vi "良率提醒告知.vi"(0 "Set Count":i32[](array[numeric]), 5 "Use Count":i32[](array[numeric])) -> (3 "String":string, 4 "OverPercentage80":bool=TRUE, 6 "Percentage 80":bool[](array[boolean]), 8 "Percentage100":bool=TRUE, 10 "ArrivePercentage100":bool[](array[boolean]))   [LabVIEW 2019]
uses:
  LLB/Commonly VI/Main Glb.vi
  LLB/Commonly VI.lvlib
panel:
  in  "Blank Button":bool
  out "Array 3":T1[](array[typedef]) items=["0_S1檢平確認氣缸_0", "1_S1檢平確認氣缸_1", "2_S1電路板檢平On次數_0", "3_S1電路板檢平On次數_1", "4_S1 電池檢平On次數_0", "5_S1 電池檢平On次數_1", "6_S1 盒蓋檢平On次數_0", "7_S1 盒蓋檢平On次數_1", "8_S2電流量測探針使用次數_0", "9_S2電流量測探針使用次數_1", "10_S2-電流量測氣缸_0", "11_S2-電流量測氣缸_1", "12_S3程式燒入 探針使用次數_0", "13_S3程式燒入 探針使用次數_1", "14_S3-程式燒入氣缸_0", "15_S3-程式燒入氣缸_1", "16_S4電壓量測探針使用次數_0", "17_S4電壓量測探針使用次數_1", "18_S4電源3V探針使用次數_0", "19_S4電源3V探針使用次數_1", "20_S4-隔離箱上蓋氣缸_0", "21_S4-隔離箱上蓋氣缸_1", "22_S4-隔離箱下蓋氣缸_0", "23_S4-隔離箱下蓋氣缸_1", "24_S4-電池電壓量測固定氣缸_0", "25_S4-電池電壓量測固定氣缸_1", "26_S4-電池電壓量測氣缸_0", "27_S4-電池電壓量測氣缸_1", "28_S4-電路板檢測氣缸_0", "29_S4-電路板檢測氣缸_1", "30_S5-電路板取料升降氣缸_0", "31_S5-電路板取料升降氣缸_1", "32_S5-電路板取料橫移氣缸_0", "33_S5-電路板取料橫移氣缸_1", "34_S5-吸真空_0", "35_S5-吸真空_1", "36_S5-破真空_0", "37_S5-破真空_1", "38_S7-焊接料件固定氣缸_0", "39_S7-焊接料件固定氣缸_1", "40_S7-焊接機清錫馬達_0", "41_S7-焊接機清錫馬達_1", "42_S10-料件翻轉區升降氣缸_0", "43_S10-料件翻轉區升降氣缸_1", "44_S10-料件翻轉區伸出氣缸_0", "45_S10-料件翻轉區伸出氣缸_1", "46_S10-料件翻轉區旋轉氣缸_0", "47_S10-料件翻轉區旋轉氣缸_1", "48_S10-料件翻轉區夾取氣缸_0", "49_S10-料件翻轉區夾取氣缸_1", "50_S10-料件橫移氣缸_0", "51_S10-料件橫移氣缸_1", "52_S10-料件吸取升降氣缸_0", "53_S10-料件吸取升降氣缸_1", "54_S10-料件放料升降氣缸_0", "55_S10-料件放料升降氣缸_1", "56_S10-吸真空_0", "57_S10-吸真空_1", "58_S10-破真空_0", "59_S10-破真空_1", "60_S11-雷射測高檢知氣缸_0", "61_S11-雷射測高檢知氣缸_1", "62_S12-熱熔升降氣缸_0", "63_S12-熱熔升降氣缸_1", "64_S12-預熱升降氣缸_0", "65_S12-預熱升降氣缸_1", "66_S12-離子槍風速調控_0", "67_S12-離子槍風速調控_1", "68_S13-吸真空_0", "69_S13-吸真空_1", "70_S13-破真空_0", "71_S13-破真空_1", "72_S13-NG蓋取料夾爪_0", "73_S13-NG蓋取料夾爪_1", "74_S13-NG蓋取料升降_0", "75_S13-NG蓋取料升降_1", "76_S13-NG電池取料升降_0", "77_S13-NG電池取料升降_1", "78_S13-NG電路板取料升降_0", "79_S13-NG電路板取料升降_1", "80_S13-NG橫移氣缸_0", "81_S13-NG橫移氣缸_1", "82_S13-NG橫移氣缸_0", "83_S13-NG橫移氣缸_1", "84_S7-焊接啟動次數_0", "85_S7-焊接啟動次數_1", "86_S12-熱熔次數_0", "87_S12-熱熔次數_1", "88_S11-雷射檢測次數_0", "89_S11-雷射檢測次數_1"]
  in  "Array 2":enum16{""}[](array[ring])
  out "cluster":T2 {"Array 4[0]" items=["0_S1檢平確認氣缸_0", "1_S1檢平確認氣缸_1", "2_S1電路板檢平On次數_0", "3_S1電路板檢平On次數_1", "4_S1 電池檢平On次數_0", "5_S1 電池檢平On次數_1", "6_S1 盒蓋檢平On次數_0", "7_S1 盒蓋檢平On次數_1", "8_S2電流量測探針使用次數_0", "9_S2電流量測探針使用次數_1", "10_S2-電流量測氣缸_0", "11_S2-電流量測氣缸_1", "12_S3程式燒入 探針使用次數_0", "13_S3程式燒入 探針使用次數_1", "14_S3-程式燒入氣缸_0", "15_S3-程式燒入氣缸_1", "16_S4電壓量測探針使用次數_0", "17_S4電壓量測探針使用次數_1", "18_S4電源3V探針使用次數_0", "19_S4電源3V探針使用次數_1", "20_S4-隔離箱上蓋氣缸_0", "21_S4-隔離箱上蓋氣缸_1", "22_S4-隔離箱下蓋氣缸_0", "23_S4-隔離箱下蓋氣缸_1", "24_S4-電池電壓量測固定氣缸_0", "25_S4-電池電壓量測固定氣缸_1", "26_S4-電池電壓量測氣缸_0", "27_S4-電池電壓量測氣缸_1", "28_S4-電路板檢測氣缸_0", "29_S4-電路板檢測氣缸_1", "30_S5-電路板取料升降氣缸_0", "31_S5-電路板取料升降氣缸_1", "32_S5-電路板取料橫移氣缸_0", "33_S5-電路板取料橫移氣缸_1", "34_S5-吸真空_0", "35_S5-吸真空_1", "36_S5-破真空_0", "37_S5-破真空_1", "38_S7-焊接料件固定氣缸_0", "39_S7-焊接料件固定氣缸_1", "40_S7-焊接機清錫馬達_0", "41_S7-焊接機清錫馬達_1", "42_S10-料件翻轉區升降氣缸_0", "43_S10-料件翻轉區升降氣缸_1", "44_S10-料件翻轉區伸出氣缸_0", "45_S10-料件翻轉區伸出氣缸_1", "46_S10-料件翻轉區旋轉氣缸_0", "47_S10-料件翻轉區旋轉氣缸_1", "48_S10-料件翻轉區夾取氣缸_0", "49_S10-料件翻轉區夾取氣缸_1", "50_S10-料件橫移氣缸_0", "51_S10-料件橫移氣缸_1", "52_S10-料件吸取升降氣缸_0", "53_S10-料件吸取升降氣缸_1", "54_S10-料件放料升降氣缸_0", "55_S10-料件放料升降氣缸_1", "56_S10-吸真空_0", "57_S10-吸真空_1", "58_S10-破真空_0", "59_S10-破真空_1", "60_S11-雷射測高檢知氣缸_0", "61_S11-雷射測高檢知氣缸_1", "62_S12-熱熔升降氣缸_0", "63_S12-熱熔升降氣缸_1", "64_S12-預熱升降氣缸_0", "65_S12-預熱升降氣缸_1", "66_S12-離子槍風速調控_0", "67_S12-離子槍風速調控_1", "68_S13-吸真空_0", "69_S13-吸真空_1", "70_S13-破真空_0", "71_S13-破真空_1", "72_S13-NG蓋取料夾爪_0", "73_S13-NG蓋取料夾爪_1", "74_S13-NG蓋取料升降_0", "75_S13-NG蓋取料升降_1", "76_S13-NG電池取料升降_0", "77_S13-NG電池取料升降_1", "78_S13-NG電路板取料升降_0", "79_S13-NG電路板取料升降_1", "80_S13-NG橫移氣缸_0", "81_S13-NG橫移氣缸_1", "82_S13-NG橫移氣缸_0", "83_S13-NG橫移氣缸_1", "84_S7-焊接啟動次數_0", "85_S7-焊接啟動次數_1", "86_S12-熱熔次數_0", "87_S12-熱熔次數_1", "88_S11-雷射檢測次數_0", "89_S11-雷射檢測次數_1"]; "Array 4[1]" items=["0_S1檢平確認氣缸_0", "1_S1檢平確認氣缸_1", "2_S1電路板檢平On次數_0", "3_S1電路板檢平On次數_1", "4_S1 電池檢平On次數_0", "5_S1 電池檢平On次數_1", "6_S1 盒蓋檢平On次數_0", "7_S1 盒蓋檢平On次數_1", "8_S2電流量測探針使用次數_0", "9_S2電流量測探針使用次數_1", "10_S2-電流量測氣缸_0", "11_S2-電流量測氣缸_1", "12_S3程式燒入 探針使用次數_0", "13_S3程式燒入 探針使用次數_1", "14_S3-程式燒入氣缸_0", "15_S3-程式燒入氣缸_1", "16_S4電壓量測探針使用次數_0", "17_S4電壓量測探針使用次數_1", "18_S4電源3V探針使用次數_0", "19_S4電源3V探針使用次數_1", "20_S4-隔離箱上蓋氣缸_0", "21_S4-隔離箱上蓋氣缸_1", "22_S4-隔離箱下蓋氣缸_0", "23_S4-隔離箱下蓋氣缸_1", "24_S4-電池電壓量測固定氣缸_0", "25_S4-電池電壓量測固定氣缸_1", "26_S4-電池電壓量測氣缸_0", "27_S4-電池電壓量測氣缸_1", "28_S4-電路板檢測氣缸_0", "29_S4-電路板檢測氣缸_1", "30_S5-電路板取料升降氣缸_0", "31_S5-電路板取料升降氣缸_1", "32_S5-電路板取料橫移氣缸_0", "33_S5-電路板取料橫移氣缸_1", "34_S5-吸真空_0", "35_S5-吸真空_1", "36_S5-破真空_0", "37_S5-破真空_1", "38_S7-焊接料件固定氣缸_0", "39_S7-焊接料件固定氣缸_1", "40_S7-焊接機清錫馬達_0", "41_S7-焊接機清錫馬達_1", "42_S10-料件翻轉區升降氣缸_0", "43_S10-料件翻轉區升降氣缸_1", "44_S10-料件翻轉區伸出氣缸_0", "45_S10-料件翻轉區伸出氣缸_1", "46_S10-料件翻轉區旋轉氣缸_0", "47_S10-料件翻轉區旋轉氣缸_1", "48_S10-料件翻轉區夾取氣缸_0", "49_S10-料件翻轉區夾取氣缸_1", "50_S10-料件橫移氣缸_0", "51_S10-料件橫移氣缸_1", "52_S10-料件吸取升降氣缸_0", "53_S10-料件吸取升降氣缸_1", "54_S10-料件放料升降氣缸_0", "55_S10-料件放料升降氣缸_1", "56_S10-吸真空_0", "57_S10-吸真空_1", "58_S10-破真空_0", "59_S10-破真空_1", "60_S11-雷射測高檢知氣缸_0", "61_S11-雷射測高檢知氣缸_1", "62_S12-熱熔升降氣缸_0", "63_S12-熱熔升降氣缸_1", "64_S12-預熱升降氣缸_0", "65_S12-預熱升降氣缸_1", "66_S12-離子槍風速調控_0", "67_S12-離子槍風速調控_1", "68_S13-吸真空_0", "69_S13-吸真空_1", "70_S13-破真空_0", "71_S13-破真空_1", "72_S13-NG蓋取料夾爪_0", "73_S13-NG蓋取料夾爪_1", "74_S13-NG蓋取料升降_0", "75_S13-NG蓋取料升降_1", "76_S13-NG電池取料升降_0", "77_S13-NG電池取料升降_1", "78_S13-NG電路板取料升降_0", "79_S13-NG電路板取料升降_1", "80_S13-NG橫移氣缸_0", "81_S13-NG橫移氣缸_1", "82_S13-NG橫移氣缸_0", "83_S13-NG橫移氣缸_1", "84_S7-焊接啟動次數_0", "85_S7-焊接啟動次數_1", "86_S12-熱熔次數_0", "87_S12-熱熔次數_1", "88_S11-雷射檢測次數_0", "89_S11-雷射檢測次數_1"]; "Array 4[2]" items=["0_S1檢平確認氣缸_0", "1_S1檢平確認氣缸_1", "2_S1電路板檢平On次數_0", "3_S1電路板檢平On次數_1", "4_S1 電池檢平On次數_0", "5_S1 電池檢平On次數_1", "6_S1 盒蓋檢平On次數_0", "7_S1 盒蓋檢平On次數_1", "8_S2電流量測探針使用次數_0", "9_S2電流量測探針使用次數_1", "10_S2-電流量測氣缸_0", "11_S2-電流量測氣缸_1", "12_S3程式燒入 探針使用次數_0", "13_S3程式燒入 探針使用次數_1", "14_S3-程式燒入氣缸_0", "15_S3-程式燒入氣缸_1", "16_S4電壓量測探針使用次數_0", "17_S4電壓量測探針使用次數_1", "18_S4電源3V探針使用次數_0", "19_S4電源3V探針使用次數_1", "20_S4-隔離箱上蓋氣缸_0", "21_S4-隔離箱上蓋氣缸_1", "22_S4-隔離箱下蓋氣缸_0", "23_S4-隔離箱下蓋氣缸_1", "24_S4-電池電壓量測固定氣缸_0", "25_S4-電池電壓量測固定氣缸_1", "26_S4-電池電壓量測氣缸_0", "27_S4-電池電壓量測氣缸_1", "28_S4-電路板檢測氣缸_0", "29_S4-電路板檢測氣缸_1", "30_S5-電路板取料升降氣缸_0", "31_S5-電路板取料升降氣缸_1", "32_S5-電路板取料橫移氣缸_0", "33_S5-電路板取料橫移氣缸_1", "34_S5-吸真空_0", "35_S5-吸真空_1", "36_S5-破真空_0", "37_S5-破真空_1", "38_S7-焊接料件固定氣缸_0", "39_S7-焊接料件固定氣缸_1", "40_S7-焊接機清錫馬達_0", "41_S7-焊接機清錫馬達_1", "42_S10-料件翻轉區升降氣缸_0", "43_S10-料件翻轉區升降氣缸_1", "44_S10-料件翻轉區伸出氣缸_0", "45_S10-料件翻轉區伸出氣缸_1", "46_S10-料件翻轉區旋轉氣缸_0", "47_S10-料件翻轉區旋轉氣缸_1", "48_S10-料件翻轉區夾取氣缸_0", "49_S10-料件翻轉區夾取氣缸_1", "50_S10-料件橫移氣缸_0", "51_S10-料件橫移氣缸_1", "52_S10-料件吸取升降氣缸_0", "53_S10-料件吸取升降氣缸_1", "54_S10-料件放料升降氣缸_0", "55_S10-料件放料升降氣缸_1", "56_S10-吸真空_0", "57_S10-吸真空_1", "58_S10-破真空_0", "59_S10-破真空_1", "60_S11-雷射測高檢知氣缸_0", "61_S11-雷射測高檢知氣缸_1", "62_S12-熱熔升降氣缸_0", "63_S12-熱熔升降氣缸_1", "64_S12-預熱升降氣缸_0", "65_S12-預熱升降氣缸_1", "66_S12-離子槍風速調控_0", "67_S12-離子槍風速調控_1", "68_S13-吸真空_0", "69_S13-吸真空_1", "70_S13-破真空_0", "71_S13-破真空_1", "72_S13-NG蓋取料夾爪_0", "73_S13-NG蓋取料夾爪_1", "74_S13-NG蓋取料升降_0", "75_S13-NG蓋取料升降_1", "76_S13-NG電池取料升降_0", "77_S13-NG電池取料升降_1", "78_S13-NG電路板取料升降_0", "79_S13-NG電路板取料升降_1", "80_S13-NG橫移氣缸_0", "81_S13-NG橫移氣缸_1", "82_S13-NG橫移氣缸_0", "83_S13-NG橫移氣缸_1", "84_S7-焊接啟動次數_0", "85_S7-焊接啟動次數_1", "86_S12-熱熔次數_0", "87_S12-熱熔次數_1", "88_S11-雷射檢測次數_0", "89_S11-雷射檢測次數_1"]; "Array 4[3]" items=["0_S1檢平確認氣缸_0", "1_S1檢平確認氣缸_1", "2_S1電路板檢平On次數_0", "3_S1電路板檢平On次數_1", "4_S1 電池檢平On次數_0", "5_S1 電池檢平On次數_1", "6_S1 盒蓋檢平On次數_0", "7_S1 盒蓋檢平On次數_1", "8_S2電流量測探針使用次數_0", "9_S2電流量測探針使用次數_1", "10_S2-電流量測氣缸_0", "11_S2-電流量測氣缸_1", "12_S3程式燒入 探針使用次數_0", "13_S3程式燒入 探針使用次數_1", "14_S3-程式燒入氣缸_0", "15_S3-程式燒入氣缸_1", "16_S4電壓量測探針使用次數_0", "17_S4電壓量測探針使用次數_1", "18_S4電源3V探針使用次數_0", "19_S4電源3V探針使用次數_1", "20_S4-隔離箱上蓋氣缸_0", "21_S4-隔離箱上蓋氣缸_1", "22_S4-隔離箱下蓋氣缸_0", "23_S4-隔離箱下蓋氣缸_1", "24_S4-電池電壓量測固定氣缸_0", "25_S4-電池電壓量測固定氣缸_1", "26_S4-電池電壓量測氣缸_0", "27_S4-電池電壓量測氣缸_1", "28_S4-電路板檢測氣缸_0", "29_S4-電路板檢測氣缸_1", "30_S5-電路板取料升降氣缸_0", "31_S5-電路板取料升降氣缸_1", "32_S5-電路板取料橫移氣缸_0", "33_S5-電路板取料橫移氣缸_1", "34_S5-吸真空_0", "35_S5-吸真空_1", "36_S5-破真空_0", "37_S5-破真空_1", "38_S7-焊接料件固定氣缸_0", "39_S7-焊接料件固定氣缸_1", "40_S7-焊接機清錫馬達_0", "41_S7-焊接機清錫馬達_1", "42_S10-料件翻轉區升降氣缸_0", "43_S10-料件翻轉區升降氣缸_1", "44_S10-料件翻轉區伸出氣缸_0", "45_S10-料件翻轉區伸出氣缸_1", "46_S10-料件翻轉區旋轉氣缸_0", "47_S10-料件翻轉區旋轉氣缸_1", "48_S10-料件翻轉區夾取氣缸_0", "49_S10-料件翻轉區夾取氣缸_1", "50_S10-料件橫移氣缸_0", "51_S10-料件橫移氣缸_1", "52_S10-料件吸取升降氣缸_0", "53_S10-料件吸取升降氣缸_1", "54_S10-料件放料升降氣缸_0", "55_S10-料件放料升降氣缸_1", "56_S10-吸真空_0", "57_S10-吸真空_1", "58_S10-破真空_0", "59_S10-破真空_1", "60_S11-雷射測高檢知氣缸_0", "61_S11-雷射測高檢知氣缸_1", "62_S12-熱熔升降氣缸_0", "63_S12-熱熔升降氣缸_1", "64_S12-預熱升降氣缸_0", "65_S12-預熱升降氣缸_1", "66_S12-離子槍風速調控_0", "67_S12-離子槍風速調控_1", "68_S13-吸真空_0", "69_S13-吸真空_1", "70_S13-破真空_0", "71_S13-破真空_1", "72_S13-NG蓋取料夾爪_0", "73_S13-NG蓋取料夾爪_1", "74_S13-NG蓋取料升降_0", "75_S13-NG蓋取料升降_1", "76_S13-NG電池取料升降_0", "77_S13-NG電池取料升降_1", "78_S13-NG電路板取料升降_0", "79_S13-NG電路板取料升降_1", "80_S13-NG橫移氣缸_0", "81_S13-NG橫移氣缸_1", "82_S13-NG橫移氣缸_0", "83_S13-NG橫移氣缸_1", "84_S7-焊接啟動次數_0", "85_S7-焊接啟動次數_1", "86_S12-熱熔次數_0", "87_S12-熱熔次數_1", "88_S11-雷射檢測次數_0", "89_S11-雷射檢測次數_1"]; "Array 4[4]" items=["0_S1檢平確認氣缸_0", "1_S1檢平確認氣缸_1", "2_S1電路板檢平On次數_0", "3_S1電路板檢平On次數_1", "4_S1 電池檢平On次數_0", "5_S1 電池檢平On次數_1", "6_S1 盒蓋檢平On次數_0", "7_S1 盒蓋檢平On次數_1", "8_S2電流量測探針使用次數_0", "9_S2電流量測探針使用次數_1", "10_S2-電流量測氣缸_0", "11_S2-電流量測氣缸_1", "12_S3程式燒入 探針使用次數_0", "13_S3程式燒入 探針使用次數_1", "14_S3-程式燒入氣缸_0", "15_S3-程式燒入氣缸_1", "16_S4電壓量測探針使用次數_0", "17_S4電壓量測探針使用次數_1", "18_S4電源3V探針使用次數_0", "19_S4電源3V探針使用次數_1", "20_S4-隔離箱上蓋氣缸_0", "21_S4-隔離箱上蓋氣缸_1", "22_S4-隔離箱下蓋氣缸_0", "23_S4-隔離箱下蓋氣缸_1", "24_S4-電池電壓量測固定氣缸_0", "25_S4-電池電壓量測固定氣缸_1", "26_S4-電池電壓量測氣缸_0", "27_S4-電池電壓量測氣缸_1", "28_S4-電路板檢測氣缸_0", "29_S4-電路板檢測氣缸_1", "30_S5-電路板取料升降氣缸_0", "31_S5-電路板取料升降氣缸_1", "32_S5-電路板取料橫移氣缸_0", "33_S5-電路板取料橫移氣缸_1", "34_S5-吸真空_0", "35_S5-吸真空_1", "36_S5-破真空_0", "37_S5-破真空_1", "38_S7-焊接料件固定氣缸_0", "39_S7-焊接料件固定氣缸_1", "40_S7-焊接機清錫馬達_0", "41_S7-焊接機清錫馬達_1", "42_S10-料件翻轉區升降氣缸_0", "43_S10-料件翻轉區升降氣缸_1", "44_S10-料件翻轉區伸出氣缸_0", "45_S10-料件翻轉區伸出氣缸_1", "46_S10-料件翻轉區旋轉氣缸_0", "47_S10-料件翻轉區旋轉氣缸_1", "48_S10-料件翻轉區夾取氣缸_0", "49_S10-料件翻轉區夾取氣缸_1", "50_S10-料件橫移氣缸_0", "51_S10-料件橫移氣缸_1", "52_S10-料件吸取升降氣缸_0", "53_S10-料件吸取升降氣缸_1", "54_S10-料件放料升降氣缸_0", "55_S10-料件放料升降氣缸_1", "56_S10-吸真空_0", "57_S10-吸真空_1", "58_S10-破真空_0", "59_S10-破真空_1", "60_S11-雷射測高檢知氣缸_0", "61_S11-雷射測高檢知氣缸_1", "62_S12-熱熔升降氣缸_0", "63_S12-熱熔升降氣缸_1", "64_S12-預熱升降氣缸_0", "65_S12-預熱升降氣缸_1", "66_S12-離子槍風速調控_0", "67_S12-離子槍風速調控_1", "68_S13-吸真空_0", "69_S13-吸真空_1", "70_S13-破真空_0", "71_S13-破真空_1", "72_S13-NG蓋取料夾爪_0", "73_S13-NG蓋取料夾爪_1", "74_S13-NG蓋取料升降_0", "75_S13-NG蓋取料升降_1", "76_S13-NG電池取料升降_0", "77_S13-NG電池取料升降_1", "78_S13-NG電路板取料升降_0", "79_S13-NG電路板取料升降_1", "80_S13-NG橫移氣缸_0", "81_S13-NG橫移氣缸_1", "82_S13-NG橫移氣缸_0", "83_S13-NG橫移氣缸_1", "84_S7-焊接啟動次數_0", "85_S7-焊接啟動次數_1", "86_S12-熱熔次數_0", "87_S12-熱熔次數_1", "88_S11-雷射檢測次數_0", "89_S11-雷射檢測次數_1"]; "Array 4[5]" items=["0_S1檢平確認氣缸_0", "1_S1檢平確認氣缸_1", "2_S1電路板檢平On次數_0", "3_S1電路板檢平On次數_1", "4_S1 電池檢平On次數_0", "5_S1 電池檢平On次數_1", "6_S1 盒蓋檢平On次數_0", "7_S1 盒蓋檢平On次數_1", "8_S2電流量測探針使用次數_0", "9_S2電流量測探針使用次數_1", "10_S2-電流量測氣缸_0", "11_S2-電流量測氣缸_1", "12_S3程式燒入 探針使用次數_0", "13_S3程式燒入 探針使用次數_1", "14_S3-程式燒入氣缸_0", "15_S3-程式燒入氣缸_1", "16_S4電壓量測探針使用次數_0", "17_S4電壓量測探針使用次數_1", "18_S4電源3V探針使用次數_0", "19_S4電源3V探針使用次數_1", "20_S4-隔離箱上蓋氣缸_0", "21_S4-隔離箱上蓋氣缸_1", "22_S4-隔離箱下蓋氣缸_0", "23_S4-隔離箱下蓋氣缸_1", "24_S4-電池電壓量測固定氣缸_0", "25_S4-電池電壓量測固定氣缸_1", "26_S4-電池電壓量測氣缸_0", "27_S4-電池電壓量測氣缸_1", "28_S4-電路板檢測氣缸_0", "29_S4-電路板檢測氣缸_1", "30_S5-電路板取料升降氣缸_0", "31_S5-電路板取料升降氣缸_1", "32_S5-電路板取料橫移氣缸_0", "33_S5-電路板取料橫移氣缸_1", "34_S5-吸真空_0", "35_S5-吸真空_1", "36_S5-破真空_0", "37_S5-破真空_1", "38_S7-焊接料件固定氣缸_0", "39_S7-焊接料件固定氣缸_1", "40_S7-焊接機清錫馬達_0", "41_S7-焊接機清錫馬達_1", "42_S10-料件翻轉區升降氣缸_0", "43_S10-料件翻轉區升降氣缸_1", "44_S10-料件翻轉區伸出氣缸_0", "45_S10-料件翻轉區伸出氣缸_1", "46_S10-料件翻轉區旋轉氣缸_0", "47_S10-料件翻轉區旋轉氣缸_1", "48_S10-料件翻轉區夾取氣缸_0", "49_S10-料件翻轉區夾取氣缸_1", "50_S10-料件橫移氣缸_0", "51_S10-料件橫移氣缸_1", "52_S10-料件吸取升降氣缸_0", "53_S10-料件吸取升降氣缸_1", "54_S10-料件放料升降氣缸_0", "55_S10-料件放料升降氣缸_1", "56_S10-吸真空_0", "57_S10-吸真空_1", "58_S10-破真空_0", "59_S10-破真空_1", "60_S11-雷射測高檢知氣缸_0", "61_S11-雷射測高檢知氣缸_1", "62_S12-熱熔升降氣缸_0", "63_S12-熱熔升降氣缸_1", "64_S12-預熱升降氣缸_0", "65_S12-預熱升降氣缸_1", "66_S12-離子槍風速調控_0", "67_S12-離子槍風速調控_1", "68_S13-吸真空_0", "69_S13-吸真空_1", "70_S13-破真空_0", "71_S13-破真空_1", "72_S13-NG蓋取料夾爪_0", "73_S13-NG蓋取料夾爪_1", "74_S13-NG蓋取料升降_0", "75_S13-NG蓋取料升降_1", "76_S13-NG電池取料升降_0", "77_S13-NG電池取料升降_1", "78_S13-NG電路板取料升降_0", "79_S13-NG電路板取料升降_1", "80_S13-NG橫移氣缸_0", "81_S13-NG橫移氣缸_1", "82_S13-NG橫移氣缸_0", "83_S13-NG橫移氣缸_1", "84_S7-焊接啟動次數_0", "85_S7-焊接啟動次數_1", "86_S12-熱熔次數_0", "87_S12-熱熔次數_1", "88_S11-雷射檢測次數_0", "89_S11-雷射檢測次數_1"]; "Array 4[6]" items=["0_S1檢平確認氣缸_0", "1_S1檢平確認氣缸_1", "2_S1電路板檢平On次數_0", "3_S1電路板檢平On次數_1", "4_S1 電池檢平On次數_0", "5_S1 電池檢平On次數_1", "6_S1 盒蓋檢平On次數_0", "7_S1 盒蓋檢平On次數_1", "8_S2電流量測探針使用次數_0", "9_S2電流量測探針使用次數_1", "10_S2-電流量測氣缸_0", "11_S2-電流量測氣缸_1", "12_S3程式燒入 探針使用次數_0", "13_S3程式燒入 探針使用次數_1", "14_S3-程式燒入氣缸_0", "15_S3-程式燒入氣缸_1", "16_S4電壓量測探針使用次數_0", "17_S4電壓量測探針使用次數_1", "18_S4電源3V探針使用次數_0", "19_S4電源3V探針使用次數_1", "20_S4-隔離箱上蓋氣缸_0", "21_S4-隔離箱上蓋氣缸_1", "22_S4-隔離箱下蓋氣缸_0", "23_S4-隔離箱下蓋氣缸_1", "24_S4-電池電壓量測固定氣缸_0", "25_S4-電池電壓量測固定氣缸_1", "26_S4-電池電壓量測氣缸_0", "27_S4-電池電壓量測氣缸_1", "28_S4-電路板檢測氣缸_0", "29_S4-電路板檢測氣缸_1", "30_S5-電路板取料升降氣缸_0", "31_S5-電路板取料升降氣缸_1", "32_S5-電路板取料橫移氣缸_0", "33_S5-電路板取料橫移氣缸_1", "34_S5-吸真空_0", "35_S5-吸真空_1", "36_S5-破真空_0", "37_S5-破真空_1", "38_S7-焊接料件固定氣缸_0", "39_S7-焊接料件固定氣缸_1", "40_S7-焊接機清錫馬達_0", "41_S7-焊接機清錫馬達_1", "42_S10-料件翻轉區升降氣缸_0", "43_S10-料件翻轉區升降氣缸_1", "44_S10-料件翻轉區伸出氣缸_0", "45_S10-料件翻轉區伸出氣缸_1", "46_S10-料件翻轉區旋轉氣缸_0", "47_S10-料件翻轉區旋轉氣缸_1", "48_S10-料件翻轉區夾取氣缸_0", "49_S10-料件翻轉區夾取氣缸_1", "50_S10-料件橫移氣缸_0", "51_S10-料件橫移氣缸_1", "52_S10-料件吸取升降氣缸_0", "53_S10-料件吸取升降氣缸_1", "54_S10-料件放料升降氣缸_0", "55_S10-料件放料升降氣缸_1", "56_S10-吸真空_0", "57_S10-吸真空_1", "58_S10-破真空_0", "59_S10-破真空_1", "60_S11-雷射測高檢知氣缸_0", "61_S11-雷射測高檢知氣缸_1", "62_S12-熱熔升降氣缸_0", "63_S12-熱熔升降氣缸_1", "64_S12-預熱升降氣缸_0", "65_S12-預熱升降氣缸_1", "66_S12-離子槍風速調控_0", "67_S12-離子槍風速調控_1", "68_S13-吸真空_0", "69_S13-吸真空_1", "70_S13-破真空_0", "71_S13-破真空_1", "72_S13-NG蓋取料夾爪_0", "73_S13-NG蓋取料夾爪_1", "74_S13-NG蓋取料升降_0", "75_S13-NG蓋取料升降_1", "76_S13-NG電池取料升降_0", "77_S13-NG電池取料升降_1", "78_S13-NG電路板取料升降_0", "79_S13-NG電路板取料升降_1", "80_S13-NG橫移氣缸_0", "81_S13-NG橫移氣缸_1", "82_S13-NG橫移氣缸_0", "83_S13-NG橫移氣缸_1", "84_S7-焊接啟動次數_0", "85_S7-焊接啟動次數_1", "86_S12-熱熔次數_0", "87_S12-熱熔次數_1", "88_S11-雷射檢測次數_0", "89_S11-雷射檢測次數_1"]; "Array 4[7]" items=["0_S1檢平確認氣缸_0", "1_S1檢平確認氣缸_1", "2_S1電路板檢平On次數_0", "3_S1電路板檢平On次數_1", "4_S1 電池檢平On次數_0", "5_S1 電池檢平On次數_1", "6_S1 盒蓋檢平On次數_0", "7_S1 盒蓋檢平On次數_1", "8_S2電流量測探針使用次數_0", "9_S2電流量測探針使用次數_1", "10_S2-電流量測氣缸_0", "11_S2-電流量測氣缸_1", "12_S3程式燒入 探針使用次數_0", "13_S3程式燒入 探針使用次數_1", "14_S3-程式燒入氣缸_0", "15_S3-程式燒入氣缸_1", "16_S4電壓量測探針使用次數_0", "17_S4電壓量測探針使用次數_1", "18_S4電源3V探針使用次數_0", "19_S4電源3V探針使用次數_1", "20_S4-隔離箱上蓋氣缸_0", "21_S4-隔離箱上蓋氣缸_1", "22_S4-隔離箱下蓋氣缸_0", "23_S4-隔離箱下蓋氣缸_1", "24_S4-電池電壓量測固定氣缸_0", "25_S4-電池電壓量測固定氣缸_1", "26_S4-電池電壓量測氣缸_0", "27_S4-電池電壓量測氣缸_1", "28_S4-電路板檢測氣缸_0", "29_S4-電路板檢測氣缸_1", "30_S5-電路板取料升降氣缸_0", "31_S5-電路板取料升降氣缸_1", "32_S5-電路板取料橫移氣缸_0", "33_S5-電路板取料橫移氣缸_1", "34_S5-吸真空_0", "35_S5-吸真空_1", "36_S5-破真空_0", "37_S5-破真空_1", "38_S7-焊接料件固定氣缸_0", "39_S7-焊接料件固定氣缸_1", "40_S7-焊接機清錫馬達_0", "41_S7-焊接機清錫馬達_1", "42_S10-料件翻轉區升降氣缸_0", "43_S10-料件翻轉區升降氣缸_1", "44_S10-料件翻轉區伸出氣缸_0", "45_S10-料件翻轉區伸出氣缸_1", "46_S10-料件翻轉區旋轉氣缸_0", "47_S10-料件翻轉區旋轉氣缸_1", "48_S10-料件翻轉區夾取氣缸_0", "49_S10-料件翻轉區夾取氣缸_1", "50_S10-料件橫移氣缸_0", "51_S10-料件橫移氣缸_1", "52_S10-料件吸取升降氣缸_0", "53_S10-料件吸取升降氣缸_1", "54_S10-料件放料升降氣缸_0", "55_S10-料件放料升降氣缸_1", "56_S10-吸真空_0", "57_S10-吸真空_1", "58_S10-破真空_0", "59_S10-破真空_1", "60_S11-雷射測高檢知氣缸_0", "61_S11-雷射測高檢知氣缸_1", "62_S12-熱熔升降氣缸_0", "63_S12-熱熔升降氣缸_1", "64_S12-預熱升降氣缸_0", "65_S12-預熱升降氣缸_1", "66_S12-離子槍風速調控_0", "67_S12-離子槍風速調控_1", "68_S13-吸真空_0", "69_S13-吸真空_1", "70_S13-破真空_0", "71_S13-破真空_1", "72_S13-NG蓋取料夾爪_0", "73_S13-NG蓋取料夾爪_1", "74_S13-NG蓋取料升降_0", "75_S13-NG蓋取料升降_1", "76_S13-NG電池取料升降_0", "77_S13-NG電池取料升降_1", "78_S13-NG電路板取料升降_0", "79_S13-NG電路板取料升降_1", "80_S13-NG橫移氣缸_0", "81_S13-NG橫移氣缸_1", "82_S13-NG橫移氣缸_0", "83_S13-NG橫移氣缸_1", "84_S7-焊接啟動次數_0", "85_S7-焊接啟動次數_1", "86_S12-熱熔次數_0", "87_S12-熱熔次數_1", "88_S11-雷射檢測次數_0", "89_S11-雷射檢測次數_1"]; "Array 4[8]" items=["0_S1檢平確認氣缸_0", "1_S1檢平確認氣缸_1", "2_S1電路板檢平On次數_0", "3_S1電路板檢平On次數_1", "4_S1 電池檢平On次數_0", "5_S1 電池檢平On次數_1", "6_S1 盒蓋檢平On次數_0", "7_S1 盒蓋檢平On次數_1", "8_S2電流量測探針使用次數_0", "9_S2電流量測探針使用次數_1", "10_S2-電流量測氣缸_0", "11_S2-電流量測氣缸_1", "12_S3程式燒入 探針使用次數_0", "13_S3程式燒入 探針使用次數_1", "14_S3-程式燒入氣缸_0", "15_S3-程式燒入氣缸_1", "16_S4電壓量測探針使用次數_0", "17_S4電壓量測探針使用次數_1", "18_S4電源3V探針使用次數_0", "19_S4電源3V探針使用次數_1", "20_S4-隔離箱上蓋氣缸_0", "21_S4-隔離箱上蓋氣缸_1", "22_S4-隔離箱下蓋氣缸_0", "23_S4-隔離箱下蓋氣缸_1", "24_S4-電池電壓量測固定氣缸_0", "25_S4-電池電壓量測固定氣缸_1", "26_S4-電池電壓量測氣缸_0", "27_S4-電池電壓量測氣缸_1", "28_S4-電路板檢測氣缸_0", "29_S4-電路板檢測氣缸_1", "30_S5-電路板取料升降氣缸_0", "31_S5-電路板取料升降氣缸_1", "32_S5-電路板取料橫移氣缸_0", "33_S5-電路板取料橫移氣缸_1", "34_S5-吸真空_0", "35_S5-吸真空_1", "36_S5-破真空_0", "37_S5-破真空_1", "38_S7-焊接料件固定氣缸_0", "39_S7-焊接料件固定氣缸_1", "40_S7-焊接機清錫馬達_0", "41_S7-焊接機清錫馬達_1", "42_S10-料件翻轉區升降氣缸_0", "43_S10-料件翻轉區升降氣缸_1", "44_S10-料件翻轉區伸出氣缸_0", "45_S10-料件翻轉區伸出氣缸_1", "46_S10-料件翻轉區旋轉氣缸_0", "47_S10-料件翻轉區旋轉氣缸_1", "48_S10-料件翻轉區夾取氣缸_0", "49_S10-料件翻轉區夾取氣缸_1", "50_S10-料件橫移氣缸_0", "51_S10-料件橫移氣缸_1", "52_S10-料件吸取升降氣缸_0", "53_S10-料件吸取升降氣缸_1", "54_S10-料件放料升降氣缸_0", "55_S10-料件放料升降氣缸_1", "56_S10-吸真空_0", "57_S10-吸真空_1", "58_S10-破真空_0", "59_S10-破真空_1", "60_S11-雷射測高檢知氣缸_0", "61_S11-雷射測高檢知氣缸_1", "62_S12-熱熔升降氣缸_0", "63_S12-熱熔升降氣缸_1", "64_S12-預熱升降氣缸_0", "65_S12-預熱升降氣缸_1", "66_S12-離子槍風速調控_0", "67_S12-離子槍風速調控_1", "68_S13-吸真空_0", "69_S13-吸真空_1", "70_S13-破真空_0", "71_S13-破真空_1", "72_S13-NG蓋取料夾爪_0", "73_S13-NG蓋取料夾爪_1", "74_S13-NG蓋取料升降_0", "75_S13-NG蓋取料升降_1", "76_S13-NG電池取料升降_0", "77_S13-NG電池取料升降_1", "78_S13-NG電路板取料升降_0", "79_S13-NG電路板取料升降_1", "80_S13-NG橫移氣缸_0", "81_S13-NG橫移氣缸_1", "82_S13-NG橫移氣缸_0", "83_S13-NG橫移氣缸_1", "84_S7-焊接啟動次數_0", "85_S7-焊接啟動次數_1", "86_S12-熱熔次數_0", "87_S12-熱熔次數_1", "88_S11-雷射檢測次數_0", "89_S11-雷射檢測次數_1"]}
  in  "Item":T1[](array[typedef])=[0, 2, 4, 6, 8, 10, 12, 14, 16, 18, 20, 22, 24, 26, 28, 30, 32, 34, 36, 38, 40, 42, 44, 46, 48, 50, 52, 54, 56, 58, 60, 62, 64, 66, 68, 70, 72, 74, 76, 78, 80, 82, 84, 86, 88] items=["0_S1檢平確認氣缸_0", "1_S1檢平確認氣缸_1", "2_S1電路板檢平On次數_0", "3_S1電路板檢平On次數_1", "4_S1 電池檢平On次數_0", "5_S1 電池檢平On次數_1", "6_S1 盒蓋檢平On次數_0", "7_S1 盒蓋檢平On次數_1", "8_S2電流量測探針使用次數_0", "9_S2電流量測探針使用次數_1", "10_S2-電流量測氣缸_0", "11_S2-電流量測氣缸_1", "12_S3程式燒入 探針使用次數_0", "13_S3程式燒入 探針使用次數_1", "14_S3-程式燒入氣缸_0", "15_S3-程式燒入氣缸_1", "16_S4電壓量測探針使用次數_0", "17_S4電壓量測探針使用次數_1", "18_S4電源3V探針使用次數_0", "19_S4電源3V探針使用次數_1", "20_S4-隔離箱上蓋氣缸_0", "21_S4-隔離箱上蓋氣缸_1", "22_S4-隔離箱下蓋氣缸_0", "23_S4-隔離箱下蓋氣缸_1", "24_S4-電池電壓量測固定氣缸_0", "25_S4-電池電壓量測固定氣缸_1", "26_S4-電池電壓量測氣缸_0", "27_S4-電池電壓量測氣缸_1", "28_S4-電路板檢測氣缸_0", "29_S4-電路板檢測氣缸_1", "30_S5-電路板取料升降氣缸_0", "31_S5-電路板取料升降氣缸_1", "32_S5-電路板取料橫移氣缸_0", "33_S5-電路板取料橫移氣缸_1", "34_S5-吸真空_0", "35_S5-吸真空_1", "36_S5-破真空_0", "37_S5-破真空_1", "38_S7-焊接料件固定氣缸_0", "39_S7-焊接料件固定氣缸_1", "40_S7-焊接機清錫馬達_0", "41_S7-焊接機清錫馬達_1", "42_S10-料件翻轉區升降氣缸_0", "43_S10-料件翻轉區升降氣缸_1", "44_S10-料件翻轉區伸出氣缸_0", "45_S10-料件翻轉區伸出氣缸_1", "46_S10-料件翻轉區旋轉氣缸_0", "47_S10-料件翻轉區旋轉氣缸_1", "48_S10-料件翻轉區夾取氣缸_0", "49_S10-料件翻轉區夾取氣缸_1", "50_S10-料件橫移氣缸_0", "51_S10-料件橫移氣缸_1", "52_S10-料件吸取升降氣缸_0", "53_S10-料件吸取升降氣缸_1", "54_S10-料件放料升降氣缸_0", "55_S10-料件放料升降氣缸_1", "56_S10-吸真空_0", "57_S10-吸真空_1", "58_S10-破真空_0", "59_S10-破真空_1", "60_S11-雷射測高檢知氣缸_0", "61_S11-雷射測高檢知氣缸_1", "62_S12-熱熔升降氣缸_0", "63_S12-熱熔升降氣缸_1", "64_S12-預熱升降氣缸_0", "65_S12-預熱升降氣缸_1", "66_S12-離子槍風速調控_0", "67_S12-離子槍風速調控_1", "68_S13-吸真空_0", "69_S13-吸真空_1", "70_S13-破真空_0", "71_S13-破真空_1", "72_S13-NG蓋取料夾爪_0", "73_S13-NG蓋取料夾爪_1", "74_S13-NG蓋取料升降_0", "75_S13-NG蓋取料升降_1", "76_S13-NG電池取料升降_0", "77_S13-NG電池取料升降_1", "78_S13-NG電路板取料升降_0", "79_S13-NG電路板取料升降_1", "80_S13-NG橫移氣缸_0", "81_S13-NG橫移氣缸_1", "82_S13-NG橫移氣缸_0", "83_S13-NG橫移氣缸_1", "84_S7-焊接啟動次數_0", "85_S7-焊接啟動次數_1", "86_S12-熱熔次數_0", "87_S12-熱熔次數_1", "88_S11-雷射檢測次數_0", "89_S11-雷射檢測次數_1"]
  out "Array":dbl[](array[numeric])
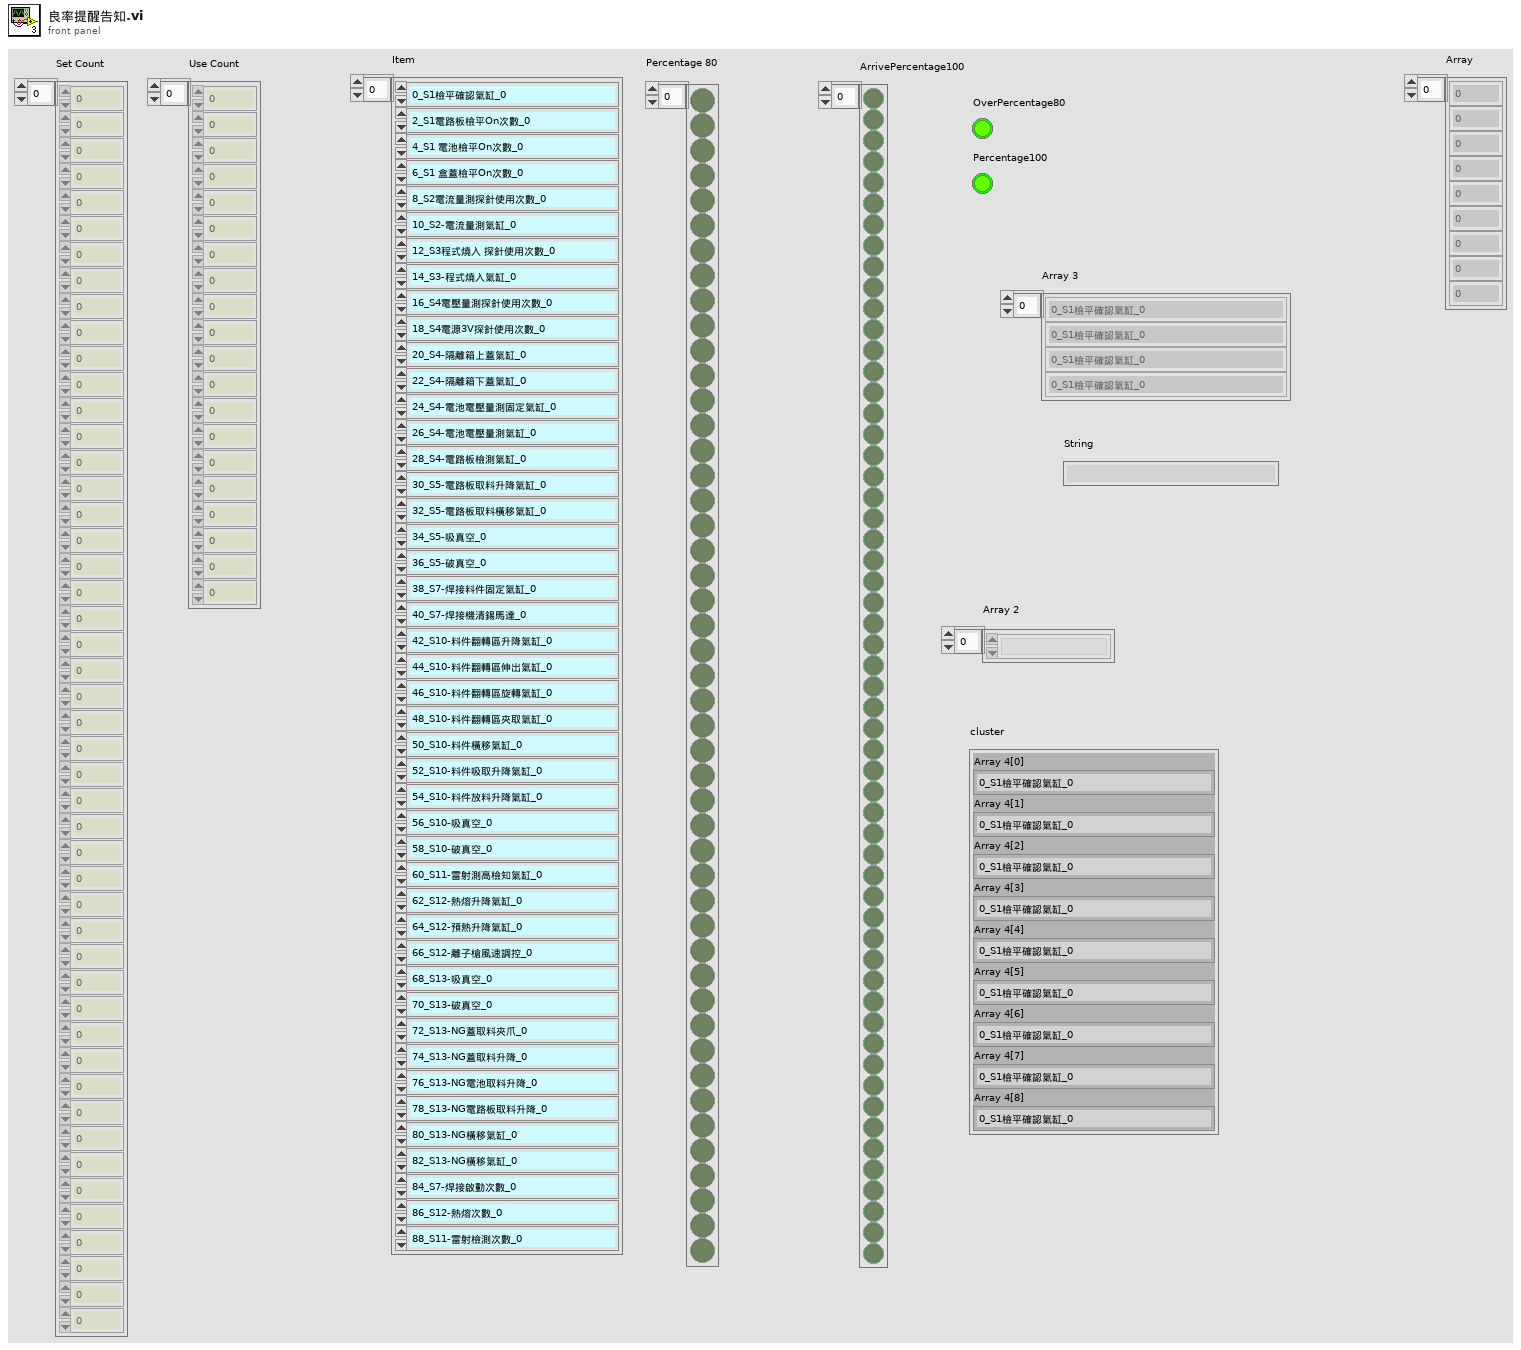
[diagram p1: front panel]
types:
  T1 = typedef "預防保養02.ctl" = u16
  T2 = cluster{"Array 4[0]":T1, "Array 4[1]":T1, "Array 4[2]":T1, "Array 4[3]":T1, "Array 4[4]":T1, "Array 4[5]":T1, "Array 4[6]":T1, "Array 4[7]":T1, "Array 4[8]":T1}
  T3 = cluster{"Item[0]":T1, "Item[1]":T1, "Item[2]":T1, "Item[3]":T1, "Item[4]":T1, "Item[5]":T1, "Item[6]":T1, "Item[7]":T1, "Item[8]":T1}
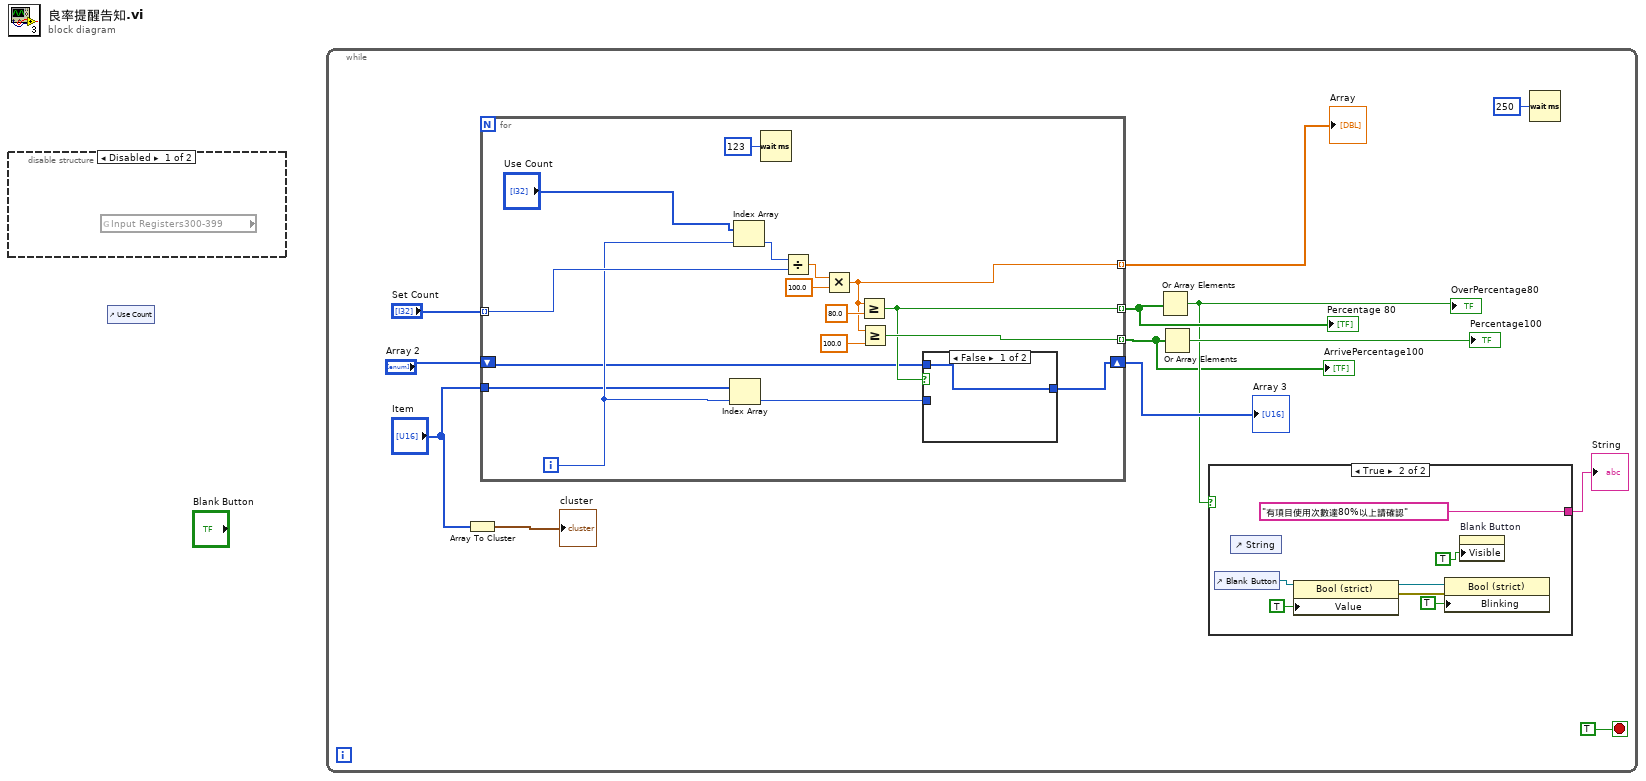
[diagram p0: block diagram]
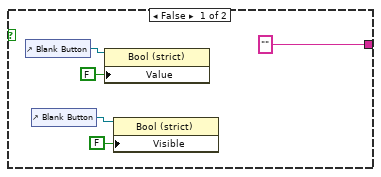
[diagram p3: hidden frame]
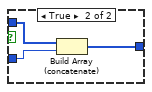
[diagram p4: hidden frame]
diagram:
  n1 = disable-structure shown="Disabled" {
    frame Disabled {
      n2 = global read "Main Glb.vi" "Input Registers300-399"() -> ()  [unwired: 1 out]
    }
    frame Enabled {
    }
  }
  n3 = control-ref of="Use Count"() -> ()  [unwired: 1 out]
  n4 = while {
    stop <- TRUE stop-if-true
    n5 = Array To Cluster(array="Item") -> (cluster=→"cluster":T3)
    n6 = for {
      tunnel: "Set Count" -> [w39] mode=indexing
      tunnel: [w35] -> w12 mode=indexing
      tunnel: [w30] -> w7 mode=indexing
      tunnel: [w33] -> w2 mode=indexing
      shift-right: [w27] -> w8
      shift-left: "Array 2" -> [w28]
      tunnel: "Item" -> [w31]
      i -> [w32]
      n7 = Index Array(array=w31, index=w32) -> (element=w29:T1)
      n8 = Index Array(array="Use Count", index=w32) -> (element=w40:i32)
      n9 = Wait (ms)(milliseconds to wait=u32 123) -> ()  [unwired: 1 out]
      n10 = Divide(x=w40, y=w39) -> (x/y=w38:dbl)
      n11 = Multiply(x=w38, y=100.0) -> (x*y=w35:dbl)
      n12 = Greater Or Equal?(x=w35, y=80.0) -> (x >= y?=w30:bool)
      n13 = Greater Or Equal?(x=w35, y=100.0) -> (x >= y?=w33:bool)
      n14 = case shown="False" w30 {
        tunnel: w29 -> [_ w44]
        tunnel: w28 -> [w42 w45]
        tunnel: [w42 w43] -> w27
        frame False {
        }
        frame True {
          n15 = Build Array (concatenate)(w45, w44) -> (w43:T1[])
        }
      }
    }
    "Array" <- w12
    "Percentage 80" <- w7
    "Array 3" <- w8
    "ArrivePercentage100" <- w2
    n16 = Or Array Elements(Boolean array=w7) -> (logical OR=w5:bool)
    "OverPercentage80" <- w5
    n17 = Or Array Elements(Boolean array=w2) -> (logical OR=→"Percentage100":bool)
    n18 = case shown="True" w5 {
      tunnel: ["" "有項目使用次數達80%以上請確認"] -> w4
      frame False {
        n19 = control-ref of="Blank Button"() -> (w17:refnum<vi>)
        n20 = control-ref of="Blank Button"() -> (w15:refnum<vi>)
        n21 = property class="Bool (strict)"(reference=w17, "Value"=FALSE) -> ()  [unwired: 1 in, 2 out]
        n22 = property class="Bool (strict)"(reference=w15, "Visible"=FALSE) -> ()  [unwired: 1 in, 2 out]
      }
      frame True {
        n23 = control-ref of="Blank Button"() -> (w23:refnum<vi>)
        n24 = control-ref of="String"() -> ()  [unwired: 1 out]
        n25 = property class="Bool (strict)"(reference=w23, "Value"=TRUE) -> (reference out=w21:refnum<vi>, error out=w20:errorcluster)  [unwired: 1 in]
        n26 = property class="Bool (strict)"(reference=w21, error in=w20, "Blinking"=TRUE) -> ()  [unwired: 2 out]
        n27 = property on="Blank Button" class="Bool (strict)"("Visible"=TRUE) -> ()  [unwired: 2 in, 2 out]
      }
    }
    "String" <- w4
    n28 = Wait (ms)(milliseconds to wait=u32 250) -> ()  [unwired: 1 out]
  }
